vi "Dynamic Call.vi"   [LabVIEW 2020]
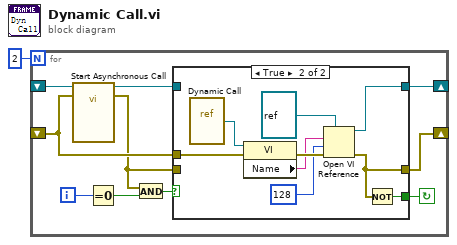
[diagram p0: block diagram]
diagram:
  n1 = for {
    N: 2 -> [_]
    shift-right: [w5] -> _
    shift-left: _ -> [w4]
    shift-right: [w6] -> _
    shift-left: _ -> [w8]
    i -> [w11]
    stop <- w2 continue-if-true
    n2 = call-by-ref "Start Asynchronous Call"(reference=w4, error in=w8) -> (reference out=w3:refnum<vi>, error out=w7:errorcluster)  [unwired: 12 in]
    n3 = Equal To 0?(x=w11) -> (x = 0?=w10:bool)
    n4 = And(x=w7, y=w10) -> (x .and. y?=w9:bool)
    n5 = case shown="True" w9 {
      tunnel: w8 -> [_ w22]
      tunnel: w7 -> [w13 _]
      tunnel: [w13 w16] -> w6
      tunnel: [w12 w18] -> w5
      tunnel: w3 -> [w12 _]
      tunnel: [_ w17] -> w2
      frame False {
      }
      frame True {
        n6 = vi-ref "Dynamic Call.vi"() -> (w15:refnum<vi>)
        n7 = property class="VI"(reference=w15, error in=w22) -> (error out=w21:errorcluster, "Name"=w20:string)  [unwired: 1 out]
        n8 = Open VI Reference(type specifier VI Refnum (for type only)=refnum<vi> refnum, vi path=w20, options=128, error in (no error)=w21) -> (vi reference=w18:refnum<vi>, error out=w16:errorcluster)  [unwired: 2 in]
        n9 = Not(x=w16) -> (.not. x?=w17:bool)
      }
    }
  }
